vi "Init Scan.vi"(8 "error in (no error)":errorcluster, 10 "Total Steps":u16, 11 "Cam_SLM_Controller in":refnum<class "Cam_SLM_Controller.lvclass">) -> (0 "error out":errorcluster, 3 "Cam_SLM_Controller out":refnum<class "Cam_SLM_Controller.lvclass">)   [LabVIEW 2023, in "Cam_SLM_controller.lvlib" / "Cam_SLM_Controller.lvclass"]
uses:
  Cam_SLM_Controller.lvclass
  Cam_SLM_Controller.lvclass/Cam_SLM_Controller.ctl
  UIs/Camera_Controller/Camera_Controller Messages/External_Acq Msg/External_Acq Msg.lvclass
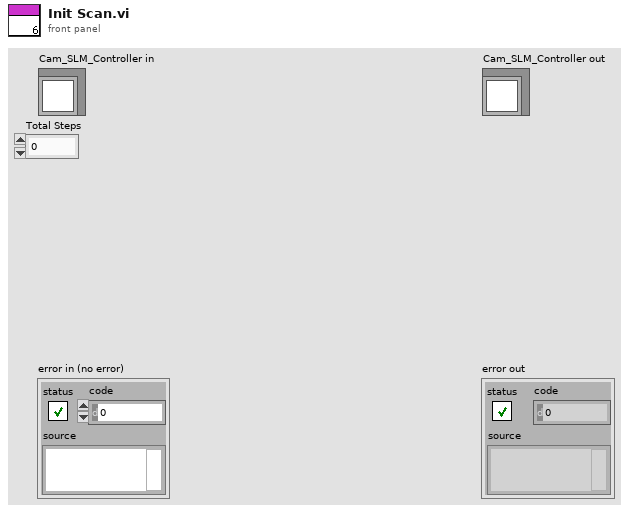
[diagram p1: front panel]
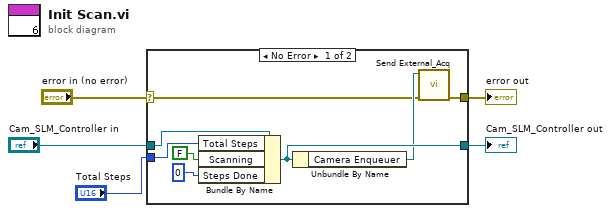
[diagram p0: block diagram]
diagram:
  n1 = case shown="No Error" "error in (no error)" {
    selector: "error in (no error)" -> [w8 w15]
    tunnel: [w7 w15] -> w4
    tunnel: [w10 w14] -> w2
    tunnel: "Cam_SLM_Controller in" -> [w13 w14]
    tunnel: "Total Steps" -> [w6 _]
    frame No Error {
      n2 = Bundle By Name(cluster=w13, "Total Steps"=w6, "Scanning"=FALSE, "Steps Done"=u16 0) -> (w10:refnum<class "Cam_SLM_Controller.lvclass">)
      n3 = Unbundle By Name(w10) -> ("Camera Enqueuer"=w9:refnum<class "Message Enqueuer.lvclass">)
      n4 = call "Send External_Acq.vi"("error in (no error)"=w8, "Message Enqueuer"=w9) -> ("error out"=w7:errorcluster)  [unwired: 8 in, 1 out]
    }
    frame Error {
    }
  }
  "error out" <- w4
  "Cam_SLM_Controller out" <- w2
